vi "Configure Output.vi"(0 "VISA resource name":refnum<visa-resource-name>, 1 "Voltage Unit (0: Volts)":i32(ring) items=["Volts", "dBm"], 2 "Frequency (50.0 Hertz)":dbl=50.0, 3 "Resistance (1900.0 Ohm)":dbl=1900.0, 5 "Output Type (0: DC Volts)":i32(ring) items=["DC Volts", "AC Volts", "DC Current", "AC Current", "DC Power", "AC Power", "Dual DC Volts", "Dual AC Volts", "Resistance"], 7 "Primary Voltage (5.0)":dbl=5.0, 9 "Secondary Voltage (5.0)":dbl=5.0, 11 "error in (no error)":errorcluster, 12 "Current (1.0 A)":dbl=1.0, 13 "Phase (0.0 Degrees)":dbl) -> (4 "VISA resource name out":refnum<visa-resource-name>, 15 "error out":errorcluster)   [LabVIEW 2012, in "Fluke 5080.lvlib"]
doc: "Configures the calibration output."
uses:
  <instrlib>/Fluke 5080/Fluke 5080.lvlib
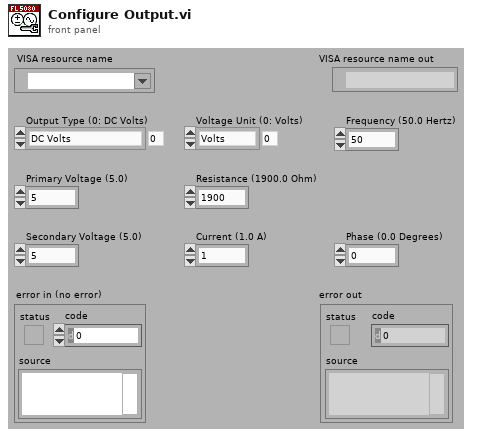
[diagram p1: front panel]
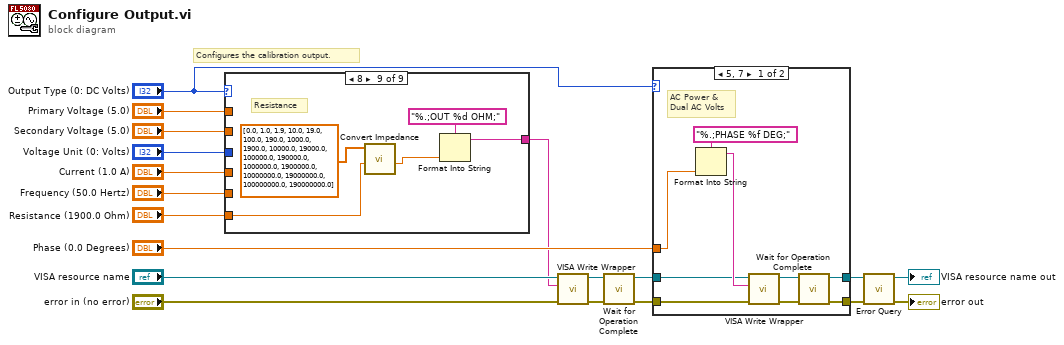
[diagram p0: block diagram]
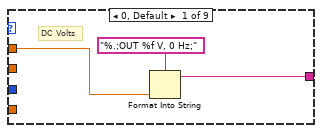
[diagram p3: hidden frame]
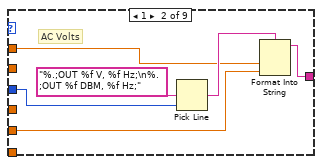
[diagram p4: hidden frame]
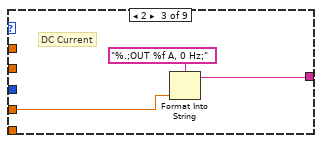
[diagram p5: hidden frame]
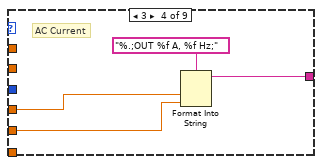
[diagram p6: hidden frame]
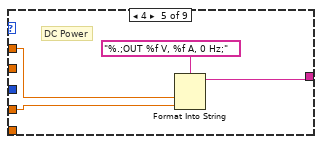
[diagram p7: hidden frame]
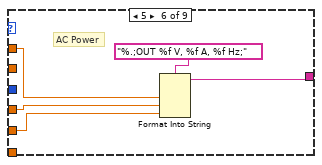
[diagram p8: hidden frame]
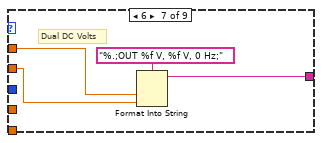
[diagram p9: hidden frame]
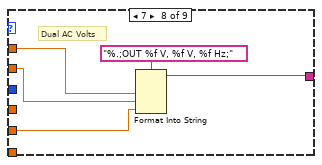
[diagram p10: hidden frame]
diagram:
  # "Configures the calibration output."
  n1 = case shown="8" "Output Type (0: DC Volts)" {
    tunnel: "Primary Voltage (5.0)" -> [w21 w25 _ _ w39 w44 w48 w52 _]
    tunnel: [w20 w24 w30 w35 w36 w40 w45 w50 w57] -> w1
    tunnel: "Voltage Unit (0: Volts)" -> [_ w28 _ _ _ _ _ _ _]
    tunnel: "Frequency (50.0 Hertz)" -> [_ w23 _ w32 _ w42 _ w49 _]
    tunnel: "Current (1.0 A)" -> [_ _ w29 w33 w38 w43 _ _ _]
    tunnel: "Secondary Voltage (5.0)" -> [_ _ _ _ _ _ w47 w51 _]
    tunnel: "Resistance (1900.0 Ohm)" -> [_ _ _ _ _ _ _ _ w56]
    frame 0, Default {
      # "DC Volts"
      n2 = Format Into String(format string="%.;OUT %f V, 0 Hz;", w21) -> (resulting string=w20:string)  [unwired: 2 in, 1 out]
    }
    frame 1 {
      # "AC Volts"
      n3 = Pick Line(multi-line string="%.;OUT %f V, %f Hz;\n%.;OUT %f DBM, %f Hz;", line index=w28) -> (output string=w26:string)  [unwired: 1 out]
      n4 = Format Into String(format string=w26, w25, w23) -> (resulting string=w24:string)  [unwired: 2 in, 1 out]
    }
    frame 2 {
      # "DC Current"
      n5 = Format Into String(format string="%.;OUT %f A, 0 Hz;", w29) -> (resulting string=w30:string)  [unwired: 2 in, 1 out]
    }
    frame 3 {
      # "AC Current"
      n6 = Format Into String(format string="%.;OUT %f A, %f Hz;" ("multi-line string"), w33, w32) -> (resulting string=w35:string)  [unwired: 2 in, 1 out]
    }
    frame 4 {
      # "DC Power"
      n7 = Format Into String(format string="%.;OUT %f V, %f A, 0 Hz;" ("multi-line string"), w39, w38) -> (resulting string=w36:string)  [unwired: 2 in, 1 out]
    }
    frame 5 {
      # "AC Power"
      n8 = Format Into String(format string="%.;OUT %f V, %f A, %f Hz;" ("multi-line string"), w44, w43, w42) -> (resulting string=w40:string)  [unwired: 2 in, 1 out]
    }
    frame 6 {
      # "Dual DC Volts"
      n9 = Format Into String(format string="%.;OUT %f V, %f V, 0 Hz;" ("multi-line string"), w48, w47) -> (resulting string=w45:string)  [unwired: 2 in, 1 out]
    }
    frame 7 {
      # "Dual AC Volts"
      n10 = Format Into String(format string="%.;OUT %f V, %f V, %f Hz;" ("multi-line string"), w52, w51, w49) -> (resulting string=w50:string)  [unwired: 2 in, 1 out]
    }
    frame 8 {
      # "Resistance"
      n11 = call <instrlib>:"Convert Impedance.vi"("Input Impedance (0 Ohm)"=w56, "Discrete Value List"=dbl[] [0.0, 1.0, 1.9, 10.0, 19.0, 100.0, 190.0, 1000.0, 1900.0, 10000.0, 19000.0, 100000.0, 190000.0, 1000000.0, 1900000.0, 10000000.0, 19000000.0, 100000000.0, 190000000.0]) -> ("Output Impedance"=w55:dbl)  [unwired: 9 out]
      n12 = Format Into String(format string="%.;OUT %d OHM;" ("multi-line string"), w55) -> (resulting string=w57:string)  [unwired: 2 in, 1 out]
    }
  }
  n13 = call <instrlib>:"VISA Write Wrapper.vi"("error in (no error)"="error in (no error)", "Write Buffer"=w1, "VISA resource name"="VISA resource name") -> ("error out"=w4:errorcluster, "VISA resource name out"=w5:refnum<visa-resource-name>)  [unwired: 6 in, 1 out]
  n14 = call <instrlib>:"Wait for Operation Complete.vi"("error in (no error)"=w4, "VISA resource name"=w5) -> ("error out"=w2:errorcluster, "VISA resource name out"=w3:refnum<visa-resource-name>)  [unwired: 8 in]
  n15 = case shown="5, 7" "Output Type (0: DC Volts)" {
    tunnel: "Phase (0.0 Degrees)" -> [w66 _]
    tunnel: w3 -> [w64 w69]
    tunnel: w2 -> [w63 w68]
    tunnel: [w60 w69] -> w7
    tunnel: [w59 w68] -> w6
    frame 5, 7 {
      # "AC Power & \nDual AC Volts"
      n16 = Format Into String(format string="%.;PHASE %f DEG;" ("multi-line string"), w66) -> (resulting string=w65:string)  [unwired: 2 in, 1 out]
      n17 = call <instrlib>:"VISA Write Wrapper.vi"("error in (no error)"=w63, "Write Buffer"=w65, "VISA resource name"=w64) -> ("error out"=w61:errorcluster, "VISA resource name out"=w62:refnum<visa-resource-name>)  [unwired: 6 in, 1 out]
      n18 = call <instrlib>:"Wait for Operation Complete.vi"("error in (no error)"=w61, "VISA resource name"=w62) -> ("error out"=w59:errorcluster, "VISA resource name out"=w60:refnum<visa-resource-name>)  [unwired: 8 in]
    }
    frame Default {
    }
  }
  n19 = call <instrlib>:"Error Query.vi"("error in (no error)"=w6, "VISA resource name"=w7) -> ("error out"=→"error out":errorcluster, "VISA resource name out"=→"VISA resource name out":refnum<visa-resource-name>)  [unwired: 8 out]
